vi "VI Server_Tree.vi"   [LabVIEW 2020]
uses:
  VI Server Toolkit LV2013.lvlib
  VI Server Libraries/VI Server_Set Controls.llb/Set 1D BOOL Control.vi
  VI Server Libraries/VI Server_Set Signaling Value.llb/Signaling_Set STR.vi
  VI Server Libraries/VI Server_SetControlValue_ArrayInputs.llb/VI Server_Set DBLs From ArrayInputs.vi
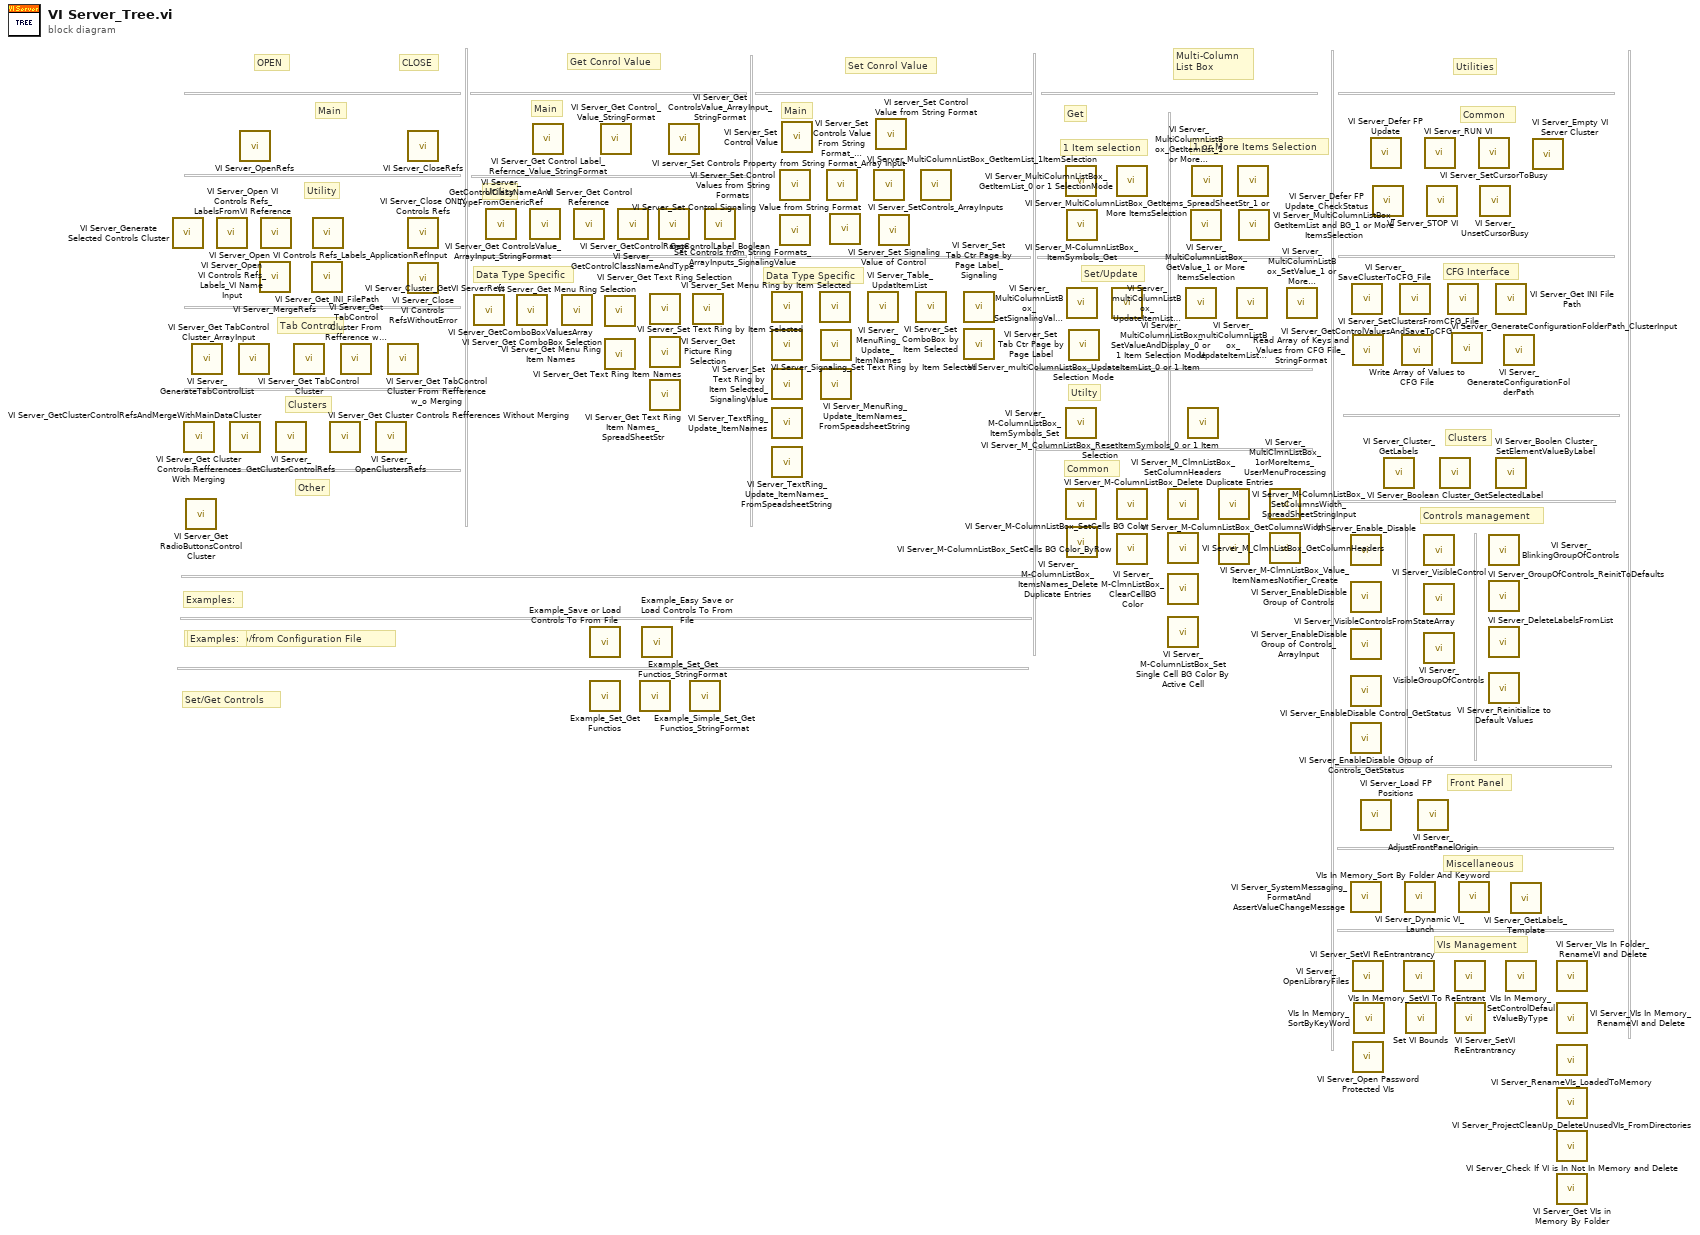
[diagram p0: block diagram]
diagram:
  # "Set/Get Controls"
  # "Save/Load to/from Configuration File"
  # "Examples:"
  # "Examples:"
  # "VIs Management"
  # "Miscellaneous"
  # "Front Panel"
  # "Controls management"
  # "Clusters"
  # "CFG Interface"
  # "Common"
  # "Utilities"
  # "Common"
  # "Utilty"
  # "Set/Update"
  # "1 or More Items Selection"
  # "1 Item selection"
  # "Get"
  # "Data Type Specific"
  # "Main"
  # "Main"
  # "Clusters"
  # "Tab Control"
  # "Utility"
  # "Main"
  # "OPEN"
  # "Other"
  # "Data Type Specific"
  # "Utility"
  # "Multi-Column\nList Box"
  # "CLOSE"
  # "Set Conrol Value"
  # "Get Conrol Value"
  n1 = call "VI Server_Generate Selected Controls Cluster.vi"() -> ()  [unwired: 10 in, 2 out]
  n2 = call "VI Server_Get Cluster Controls Refferences With Merging.vi"() -> ()  [unwired: 8 in, 4 out]
  n3 = call "VI Server_Get RadioButtonsControl Cluster.vi"() -> ()  [unwired: 9 in, 3 out]
  n4 = call "VI Server_GenerateTabControlList.vi"() -> ()  [unwired: 9 in, 3 out]
  n5 = call "VI Server_Open VI Controls Refs_Labels_VI Name Input.vi"() -> ()  [unwired: 10 in, 2 out]
  n6 = call "VI Server_GetClusterControlRefsAndMergeWithMainDataCluster.vi"() -> ()  [unwired: 8 in, 4 out]
  n7 = call "VI Server_Get TabControl Cluster_ArrayInput.vi"() -> ()  [unwired: 10 in, 2 out]
  n8 = call "VI Server_OpenRefs.vi"() -> ()  [unwired: 10 in, 2 out]
  n9 = call "VI Server_MergeRefs.vi"() -> ()  [unwired: 10 in, 2 out]
  n10 = call "VI Server_Open VI Controls Refs_LabelsFromVI Reference.vi"() -> ()  [unwired: 10 in, 2 out]
  n11 = call "VI Server_GetClusterControlRefs.vi"() -> ()  [unwired: 8 in, 4 out]
  n12 = call "VI Server_Get TabControl Cluster.vi"() -> ()  [unwired: 10 in, 2 out]
  n13 = call "VI Server_Get_INI_FilePath.vi"() -> ()  [unwired: 9 in, 3 out]
  n14 = call "VI Server_Open VI Controls Refs_Labels_ApplicationRefInput.vi"() -> ()  [unwired: 10 in, 2 out]
  n15 = call "VI Server_Get Cluster Controls Refferences Without Merging.vi"() -> ()  [unwired: 9 in, 3 out]
  n16 = call "VI Server_Get TabControl Cluster From Refference w Merging.vi"() -> ()  [unwired: 10 in, 2 out]
  n17 = call "VI Server_OpenClustersRefs.vi"() -> ()  [unwired: 10 in, 2 out]
  n18 = call "VI Server_Get TabControl Cluster From Refference w_o Merging.vi"() -> ()  [unwired: 9 in, 3 out]
  n19 = call "VI Server_CloseRefs.vi"() -> ()  [unwired: 11 in, 1 out]
  n20 = call "VI Server_Close ONLY Controls Refs.vi"() -> ()  [unwired: 11 in, 1 out]
  n21 = call "VI Server_Close VI Controls RefsWithoutError.vi"() -> ()  [unwired: 11 in, 1 out]
  n22 = call "VI Server_Cluster_GetVI ServerRefs.vi"() -> ()  [unwired: 9 in, 3 out]
  n23 = call "VI Server_GetControlClassNameAndTypeFromGenericRef.vi"() -> ()  [unwired: 8 in, 4 out]
  n24 = call "VI Server_Get ComboBox Selection.vi"() -> ()  [unwired: 6 in, 6 out]
  n25 = call "VI Server_Get ControlsValue_ArrayInput_StringFormat.vi"() -> ()  [unwired: 7 in, 5 out]
  n26 = call "VI Server_Get Control Label_Refernce_Value_StringFormat.vi"() -> ()  [unwired: 9 in, 3 out]
  n27 = call "VI Server_GetComboBoxValuesArray.vi"() -> ()  [unwired: 7 in, 5 out]
  n28 = call "VI Server_Get Control Reference.vi"() -> ()  [unwired: 8 in, 4 out]
  n29 = call "Example_Save or Load Controls To From File.vi"() -> ()  [unwired: 12 in]
  n30 = call "Example_Set_Get Functios.vi"() -> ()  [unwired: 12 in]
  n31 = call "VI Server_Get Control_Value_StringFormat.vi"() -> ()  [unwired: 8 in, 4 out]
  n32 = call "VI Server_Get Menu Ring Selection.vi"() -> ()  [unwired: 6 in, 6 out]
  n33 = call "VI Server_Get Menu Ring Item Names.vi"() -> ()  [unwired: 6 in, 6 out]
  n34 = call "VI Server_GetControlClassNameAndType.vi"() -> ()  [unwired: 8 in, 4 out]
  n35 = call "Example_Set_Get Functios_StringFormat.vi"() -> ()  [unwired: 12 in]
  n36 = call "Example_Easy Save or Load Controls To From File.vi"() -> ()  [unwired: 12 in]
  n37 = call "VI Server_Get Text Ring Selection.vi"() -> ()  [unwired: 6 in, 6 out]
  n38 = call "VI Server_Get Text Ring Item Names.vi"() -> ()  [unwired: 6 in, 6 out]
  n39 = call "VI Server_Get Text Ring Item Names_SpreadSheetStr.vi"() -> ()  [unwired: 6 in, 6 out]
  n40 = call "VI Server_GetControlRange.vi"() -> ()  [unwired: 10 in, 2 out]
  n41 = call "VI Server_Get ControlsValue_ArrayInput_StringFormat.vi"() -> ()  [unwired: 7 in, 5 out]
  n42 = call "Example_Simple_Set_Get Functios_StringFormat.vi"() -> ()  [unwired: 12 in]
  n43 = call "VI Server_Get Picture Ring Selection.vi"() -> ()  [unwired: 6 in, 6 out]
  n44 = call "GetControlLabel_Boolean.vi"() -> ()  [unwired: 10 in, 2 out]
  n45 = call "VI Server_Set Text Ring by Item Selected.vi"() -> ()  [unwired: 9 in, 3 out]
  n46 = call "VI Server_Signaling_Set Text Ring by Item Selected.vi"() -> ()  [unwired: 9 in, 3 out]
  n47 = call "VI Server_Set Text Ring by Item Selected_SignalingValue.vi"() -> ()  [unwired: 9 in, 3 out]
  n48 = call "VI Server_TextRing_Update_ItemNames.vi"() -> ()  [unwired: 9 in, 3 out]
  n49 = call "VI Server_TextRing_Update_ItemNames_FromSpeadsheetString.vi"() -> ()  [unwired: 9 in, 3 out]
  n50 = call "VI Server_Set Control Values from String Formats.vi"() -> ()  [unwired: 9 in, 3 out]
  n51 = call "Set Controls from String Formats_ArrayInputs_SignalingValue.vi"() -> ()  [unwired: 10 in, 2 out]
  n52 = call-poly "VI Server_Set Control Value.vi"() -> ()  [unwired: 9 in, 3 out]
  n53 = call "VI Server_Set Menu Ring by Item Selected.vi"() -> ()  [unwired: 9 in, 3 out]
  n54 = call "VI Server_MenuRing_Update_ItemNames.vi"() -> ()  [unwired: 9 in, 3 out]
  n55 = call "VI Server_MenuRing_Update_ItemNames_FromSpeadsheetString.vi"() -> ()  [unwired: 8 in, 4 out]
  n56 = call "VI Server_Set Controls Value From String Format_ArrayInputs.vi"() -> ()  [unwired: 10 in, 2 out]
  n57 = call "VI Server_Set Control Signaling Value from String Format.vi"() -> ()  [unwired: 10 in, 2 out]
  n58 = call "VI Server_Table_UpdatItemList.vi"() -> ()  [unwired: 9 in, 3 out]
  n59 = call "VI server_Set Controls Property from String Format_Array Input.vi"() -> ()  [unwired: 10 in, 2 out]
  n60 = call "VI server_Set Control Value from String Format.vi"() -> ()  [unwired: 9 in, 3 out]
  n61 = call-poly "VI Server_Set Signaling Value of Control.vi"() -> ()  [unwired: 9 in, 3 out]
  n62 = call "VI Server_Set ComboBox by Item Selected.vi"() -> ()  [unwired: 9 in, 3 out]
  n63 = call-poly "VI Server_SetControls_ArrayInputs.vi"() -> ()  [unwired: 9 in, 3 out]
  n64 = call "VI Server_Set Tab Ctr Page by Page Label_Signaling.vi"() -> ()  [unwired: 10 in, 2 out]
  n65 = call "VI Server_Set Tab Ctr Page by Page Label.vi"() -> ()  [unwired: 10 in, 2 out]
  n66 = call "VI Server_MultiColumnListBox_GetItemList_1ItemSelection.vi"() -> ()  [unwired: 6 in, 6 out]
  n67 = call "VI Server_M-ColumnListBox_ItemSymbols_Set.vi"() -> ()  [unwired: 9 in, 3 out]
  n68 = call "VI Server_M-ColumnListBox_Delete Duplicate Entries.vi"() -> ()  [unwired: 9 in, 3 out]
  n69 = call "VI Server_M-ColumnListBox_ItemSymbols_Get.vi"() -> ()  [unwired: 8 in, 4 out]
  n70 = call "VI Server_MultiColumnListBox_SetSignalingValueAndDisplay_0 or 1 Selection.vi"() -> ()  [unwired: 10 in, 2 out]
  n71 = call "VI Server_M-ColumnListBox_ItemsNames_Delete Duplicate Entries.vi"() -> ()  [unwired: 10 in, 2 out]
  n72 = call "VI Server_multiColumnListBox_UpdateItemList_0 or 1 Item Selection Mode.vi"() -> ()  [unwired: 9 in, 3 out]
  n73 = call "VI Server_MultiColumnListBox_SetValueAndDisplay_0 or 1 Item Selection Mode.vi"() -> ()  [unwired: 10 in, 2 out]
  n74 = call "VI Server_MultiColumnListBox_GetItemList_0 or 1 SelectionMode.vi"() -> ()  [unwired: 6 in, 6 out]
  n75 = call "VI Server_M-ColumnListBox_SetCells BG Color.vi"() -> ()  [unwired: 10 in, 2 out]
  n76 = call "VI Server_M-ColumnListBox_SetCells BG Color_ByRow.vi"() -> ()  [unwired: 10 in, 2 out]
  n77 = call "VI Server_M_ClmnListBox_SetColumnHeaders.vi"() -> ()  [unwired: 9 in, 3 out]
  n78 = call "VI Server_M_ClmnListBox_GetColumnHeaders.vi"() -> ()  [unwired: 7 in, 5 out]
  n79 = call "VI Server_M-ClmnListBox_ClearCellBG Color.vi"() -> ()  [unwired: 10 in, 2 out]
  n80 = call "VI Server_M-ColumnListBox_Set Single Cell BG Color By Active Cell.vi"() -> ()  [unwired: 10 in, 2 out]
  n81 = call "VI Server_multiColumnListBox_UpdateItemList_1 or More Items Selection.vi"() -> ()  [unwired: 8 in, 4 out]
  n82 = call "VI Server_M_ColumnListBox_ResetItemSymbols_0 or 1 Item Selection.vi"() -> ()  [unwired: 9 in, 3 out]
  n83 = call "VI Server_MultiColumnListBox_GetValue_1 or More ItemsSelection.vi"() -> ()  [unwired: 6 in, 6 out]
  n84 = call "VI Server_MultiColumnListBox_GetItemList_1 or More ItemsSelection.vi"() -> ()  [unwired: 6 in, 6 out]
  n85 = call "VI Server_M-ColumnListBox_SetColumnsWidth_SpreadSheetStringInput.vi"() -> ()  [unwired: 9 in, 3 out]
  n86 = call "VI Server_M-ColumnListBox_GetColumnsWidth.vi"() -> ()  [unwired: 8 in, 4 out]
  n87 = call "VI Server_multiColumnListBox_UpdateItemList_SpreadSheetStr_1 or More Items Selection.vi"() -> ()  [unwired: 8 in, 4 out]
  n88 = call "VI Server_MultiColumnListBox_GetItems_SpreadSheetStr_1 or More ItemsSelection.vi"() -> ()  [unwired: 6 in, 6 out]
  n89 = call "VI Server_MultiColumnListBox_GetItemList and BG_1 or More ItemsSelection.vi"() -> ()  [unwired: 5 in, 7 out]
  n90 = call "VI Server_MultiClmnListBox_1orMoreItems_UserMenuProcessing.vi"() -> ()  [unwired: 11 in, 1 out]
  n91 = call "VI Server_M-ClmnListBox_Value_ItemNamesNotifier_Create.vi"() -> ()  [unwired: 10 in, 2 out]
  n92 = call "VI Server_MultiColumnListBox_SetValue_1 or More ItemsSelection.vi"() -> ()  [unwired: 7 in, 5 out]
  n93 = call "VI Server_Enable_Disable.vi"() -> ()  [unwired: 9 in, 3 out]
  n94 = call "VI Server_EnableDisable Group of Controls.vi"() -> ()  [unwired: 9 in, 3 out]
  n95 = call "VI Server_EnableDisable Group of Controls_ArrayInput.vi"() -> ()  [unwired: 10 in, 2 out]
  n96 = call "VI Server_EnableDisable Control_GetStatus.vi"() -> ()  [unwired: 9 in, 3 out]
  n97 = call "VI Server_EnableDisable Group of Controls_GetStatus.vi"() -> ()  [unwired: 9 in, 3 out]
  n98 = call "VI Server_SystemMessaging_FormatAnd AssertValueChangeMessage.vi"() -> ()  [unwired: 9 in, 3 out]
  n99 = call "VI Server_GetControlValuesAndSaveToCFG.vi"() -> ()  [unwired: 8 in, 4 out]
  n100 = call "Read Array of Keys and Values from CFG File_StringFormat.vi"() -> ()  [unwired: 10 in, 2 out]
  n101 = call "VI Server_OpenLibraryFiles.vi"() -> ()  [unwired: 1 in]
  n102 = call "VI Server_Open Password Protected VIs.vi"() -> ()  [unwired: 1 in]
  n103 = call "VIs In Memory_SortByKeyWord.vi"() -> ()  [unwired: 11 in, 1 out]
  n104 = call "VI Server_Load FP Positions.vi"() -> ()  [unwired: 10 in, 2 out]
  n105 = call "VI Server_Defer FP Update.vi"() -> ()  [unwired: 10 in, 2 out]
  n106 = call "VI Server_Defer FP Update_CheckStatus.vi"() -> ()  [unwired: 9 in, 3 out]
  n107 = call "VI Server_Cluster_GetLabels.vi"() -> ()  [unwired: 9 in, 3 out]
  n108 = call "VI Server_SaveClusterToCFG_File.vi"() -> ()  [unwired: 9 in, 2 out]
  n109 = call "Write Array of Values to CFG File.vi"() -> ()  [unwired: 10 in, 2 out]
  n110 = call "VI Server_SetVI ReEntrantrancy.vi"() -> ()  [unwired: 1 in]
  n111 = call "VI Server_Dynamic VI_Launch.vi"() -> ()  [unwired: 10 in, 2 out]
  n112 = call "Set VI Bounds.vi"() -> ()  [unwired: 10 in, 2 out]
  n113 = call "VI Server_AdjustFrontPanelOrigin.vi"() -> ()  [unwired: 11 in, 1 out]
  n114 = call "VI Server_VisibleControl.vi"() -> ()  [unwired: 10 in, 2 out]
  n115 = call "VI Server_VisibleControlsFromStateArray.vi"() -> ()  [unwired: 10 in, 2 out]
  n116 = call "VI Server_VisibleGroupOfControls.vi"() -> ()  [unwired: 9 in, 3 out]
  n117 = call "VI Server_RUN VI.vi"() -> ()  [unwired: 11 in, 1 out]
  n118 = call "VI Server_STOP VI.vi"() -> ()  [unwired: 11 in, 1 out]
  n119 = call "VI Server_Boolean Cluster_GetSelectedLabel.vi"() -> ()  [unwired: 9 in, 3 out]
  n120 = call "VI Server_SetClustersFromCFG_File.vi"() -> ()  [unwired: 9 in, 2 out]
  n121 = call "VI Server_GenerateConfigurationFolderPath_ClusterInput.vi"() -> ()  [unwired: 13 in, 3 out]
  n122 = call "VIs In Memory_SetVI To ReEntrant.vi"() -> ()  [unwired: 1 in]
  n123 = call "VI Server_SetVI ReEntrantrancy.vi"() -> ()  [unwired: 1 in]
  n124 = call "VIs In Memory_Sort By Folder And Keyword.vi"() -> ()  [unwired: 10 in, 2 out]
  n125 = call "VI Server_SetCursorToBusy.vi"() -> ()  [unwired: 10 in, 2 out]
  n126 = call "VI Server_UnsetCursorBusy.vi"() -> ()  [unwired: 10 in, 2 out]
  n127 = call "VI Server_BlinkingGroupOfControls.vi"() -> ()  [unwired: 10 in, 2 out]
  n128 = call "VI Server_GroupOfControls_ReinitToDefaults.vi"() -> ()  [unwired: 10 in, 2 out]
  n129 = call "VI Server_DeleteLabelsFromList.vi"() -> ()  [unwired: 11 in, 1 out]
  n130 = call "VI Server_Reinitialize to Default Values.vi"() -> ()  [unwired: 10 in, 2 out]
  n131 = call "VI Server_Get INI File Path.vi"() -> ()  [unwired: 8 in, 3 out]
  n132 = call "VI Server_Boolen Cluster_SetElementValueByLabel.vi"() -> ()  [unwired: 10 in, 2 out]
  n133 = call "VI Server_GenerateConfigurationFolderPath.vi"() -> ()  [unwired: 14 in, 2 out]
  n134 = call "VIs In Memory_SetControlDefaultValueByType.vi"() -> ()  [unwired: 1 in]
  n135 = call "VI Server_GetLabels_Template.vi"() -> ()  [unwired: 12 in]
  n136 = call "VI Server_Empty VI Server Cluster.vi"() -> ()  [unwired: 7 in, 1 out]
  n137 = call "VI Server_VIs In Folder_RenameVI and Delete.vi"() -> ()  [unwired: 10 in, 2 out]
  n138 = call "VI Server_VIs In Memory_RenameVI and Delete.vi"() -> ()  [unwired: 10 in, 2 out]
  n139 = call "VI Server_RenameVIs_LoadedToMemory.vi"() -> ()  [unwired: 12 in]
  n140 = call "VI Server_ProjectCleanUp_DeleteUnusedVIs_FromDirectories.vi"() -> ()  [unwired: 12 in]
  n141 = call "VI Server_Check If VI is In Not In Memory and Delete.vi"() -> ()  [unwired: 9 in, 3 out]
  n142 = call "VI Server_Get VIs in Memory By Folder.vi"() -> ()  [unwired: 8 in, 4 out]
